vi "Simple navdata with gotoxy.vi"() -> ()   [LabVIEW 2014]
doc: "Very simple example showing how to use the base VIs to control the AR Drone and receive and display navigation data."
uses:
  <vilib>/LVH/AR Drone Toolkit/Decode NavData/Typedefs/NavData Demo.ctl
  <vilib>/LVH/AR Drone Toolkit/AR Drone.lvlib
  <vilib>/ptbypt/NI_PtbyPt.lvlib
panel:
  out "Control Cluster 2":T1
  out "XY Graph":cluster{"Y":dbl[], "Y":dbl[]}[](graph)
  in  "stop 2":bool
  in  "Emergency Landing 2":bool
  in  "Take Off/Land 2":bool
  in  "Hover 2":bool
  in  "Y goal":dbl
  in  "X goal":dbl
  out "Battery Remaining":dbl(slide) scale=0.0..100.0
  out "NavData Out":T2
  in  "Control Cluster":T1 {"Yaw Speed" scale=-1.0..1.0; "Vertical Speed" scale=-1.0..1.0; "Pitch" scale=-1.0..1.0; "Roll" scale=-1.0..1.0}
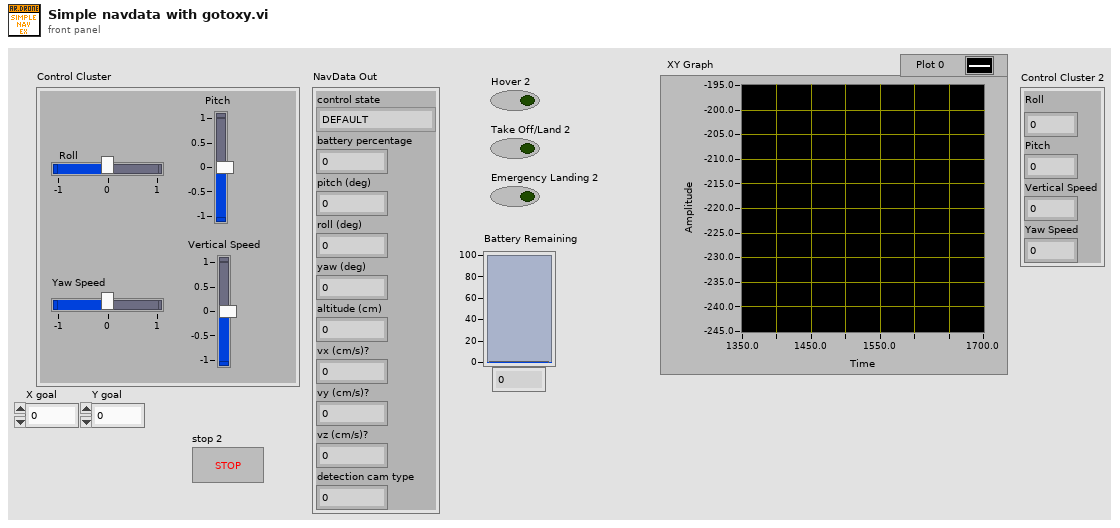
[diagram p1: front panel]
types:
  T1 = cluster{"Roll":sgl, "Pitch":sgl, "Vertical Speed":sgl, "Yaw Speed":sgl}
  T2 = typedef "AR Drone.lvlib/NavData Demo.ctl" = cluster{"control state":enum32{"DEFAULT", "INIT", "LANDING", "FLYING", "HOVERING", "TEST", "TRANS_TAKEOFF", "TRANS_GOTOFIX", "TRANS_LANDING"}, "battery percentage":u32, "pitch (deg)":sgl, "roll (deg)":sgl, "yaw (deg)":sgl, "altitude (cm)":u32, "vx (cm/s)?":sgl, "vy (cm/s)?":sgl, "vz (cm/s)?":sgl, "detection cam type":u32}
  T3 = typedef "AR Drone.lvlib/AR Drone Resource.ctl" = cluster{"UDP Control Connection":refnum<k16>, "UDP NavData Connection":refnum<k16>, "UDP Video Connection (Drone 1.0)":refnum<k16>, "TCP Video Connection (Drone 2.0)":refnum<k5>, "TCP Control Port Connection":refnum<k5>, "Drone IP address":string, "Drone Command Port":u16, "Drone NavData Port":u16, "Drone Vid Stream Port":u16, "Drone TCP Control Port":u16, "Home IP address":string, "Home Command Port":u16, "Home NavData Port":u16, "Home Vid Stream Port":u16, "Drone Version":i32}
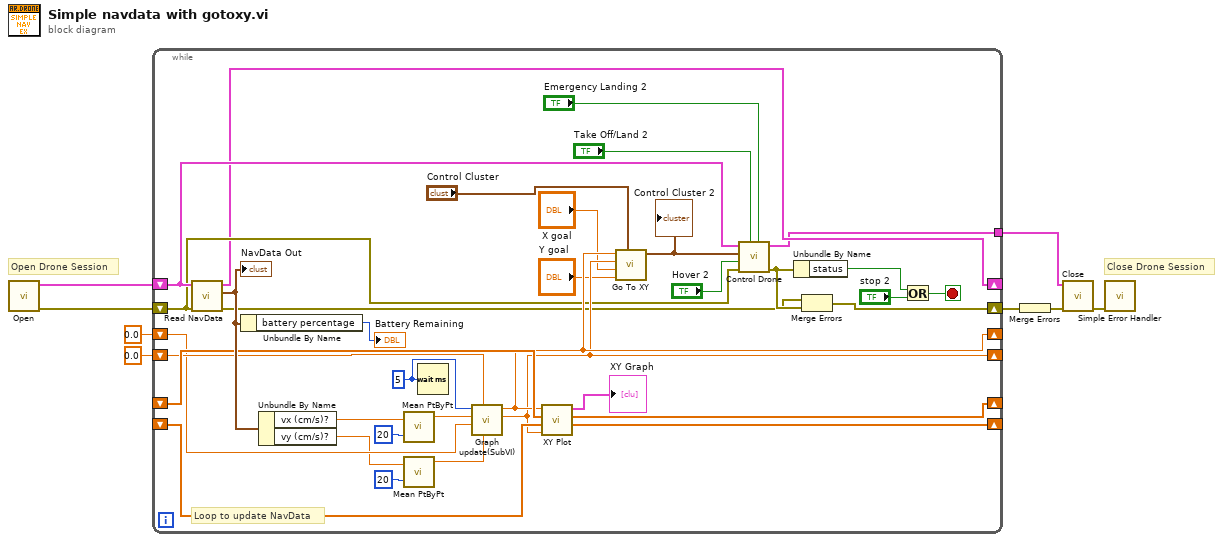
[diagram p0: block diagram]
diagram:
  # "Close Drone Session"
  # "Open Drone Session"
  n1 = call <vilib>:"Open.vi"() -> ("error out"=w7:errorcluster, "AR Drone Resource"=w8:T3)  [unwired: 10 in]
  n2 = while {
    shift-right: [w22] -> _
    shift-left: w8 -> [w25]
    shift-right: [w19] -> w2
    shift-left: w7 -> [w24]
    shift-right: [w40] -> _
    shift-left: _ -> [w37]
    shift-right: [w39] -> _
    shift-left: _ -> [w38]
    shift-right: [w34] -> _
    shift-left: 0.0 ("Numeric 3") -> [w35]
    shift-right: [w33] -> _
    shift-left: 0.0 ("Numeric out") -> [w36]
    tunnel: [w17] -> w1
    stop <- w23 stop-if-true
    w42 = u32 5 ("milliseconds to wait")
    # "Loop to update NavData"
    n3 = call <vilib>:"Read NavData.vi"("error in (no error)"=w24, "AR Drone Resource"=w25) -> ("error out"=w20:errorcluster, "NavData Out"=w41:T2, "AR Drone Resource Out"=w22:T3)  [unwired: 7 in]
    "NavData Out" <- w41
    n4 = Unbundle By Name(w41) -> ("battery percentage"=→"Battery Remaining":u32)
    n5 = Unbundle By Name(w41) -> ("vx (cm/s)?"=w16:sgl, "vy (cm/s)?"=w12:sgl)
    n6 = call <vilib>:"Mean PtByPt.vi"("x"=w16, "sample length"=20) -> ("mean"=w14:dbl)  [unwired: 2 in, 1 out]
    n7 = call <vilib>:"Mean PtByPt.vi"("x"=w12, "sample length"=20) -> ("mean"=w11:dbl)  [unwired: 2 in, 1 out]
    n8 = Wait (ms)(milliseconds to wait=w42) -> ()  [unwired: 1 out]
    n9 = call "Graph update(SubVI).vi"("vy (cm/s)?"=w11, "Numeric 4"=w36, "Numeric in"=w35, "vx (cm/s)?"=w14, "milliseconds to wait"=w42) -> ("Numeric out"=w33:dbl, "Numeric 3"=w34:dbl)  [unwired: 5 in]
    n10 = call "XY Plot.vi"("X"=w34, "X array"=w37, "Y array"=w38, "Y"=w33) -> ("XY Graph"=→"XY Graph":cluster{"Y":dbl[], "Y":dbl[]}[], "X array"=w40:dbl[], "Y array"=w39:dbl[])  [unwired: 2 in, 1 out]
    n11 = call "Go To XY.vi"("Control Cluster"="Control Cluster", "Y goal"="Y goal", "X goal"="X goal", "Y current"=w33, "X current"=w34) -> ("Control Cluster"=w9:T1)  [unwired: 6 in]
    "Control Cluster 2" <- w9
    n12 = call <vilib>:"Control Drone.vi"("Emergency Landing"="Emergency Landing 2", "Takeoff/Land"="Take Off/Land 2", "error in (no error)"=w24, "Hover"="Hover 2", "Control Cluster"=w9, "AR Drone Resource"=w25) -> ("error out"=w21:errorcluster, "AR Drone Resource Out"=w17:T3)  [unwired: 4 in]
    n13 = Unbundle By Name(w21) -> ("status"=w27:bool)
    n14 = Merge Errors(w20, w21) -> (w19:errorcluster)
    n15 = Or(x=w27, y="stop 2") -> (x .or. y?=w23:bool)
  }
  n16 = Merge Errors(w2) -> (w6:errorcluster)
  n17 = call <vilib>:"Close.vi"("error in (no error)"=w6, "AR Drone Resource"=w1) -> ("error out"=w5:errorcluster)  [unwired: 9 in]
  n18 = call <vilib>:"Simple Error Handler.vi"("error in (no error)"=w5) -> ()  [unwired: 4 in, 5 out]
